vi "WildDrive.vi"(8 "Super Turn":bool, 9 "Turn":dbl, 11 "Speed":dbl) -> (1 "Right Side Power":dbl, 3 "Left Side Power":dbl)   [LabVIEW 2018]
panel:
  in  "Manual Feed Forward (Turn)":dbl
  in  "Manual Feed Forward (speed)":dbl
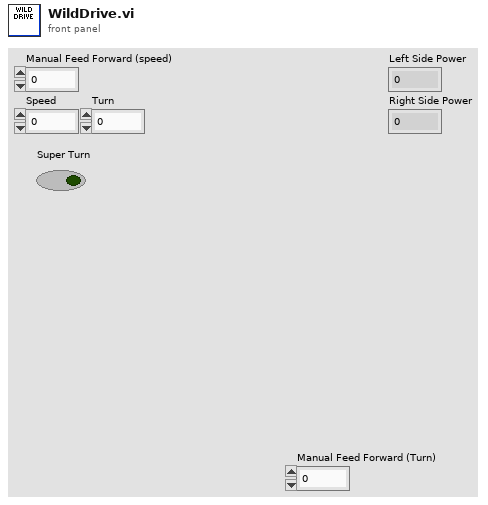
[diagram p1: front panel]
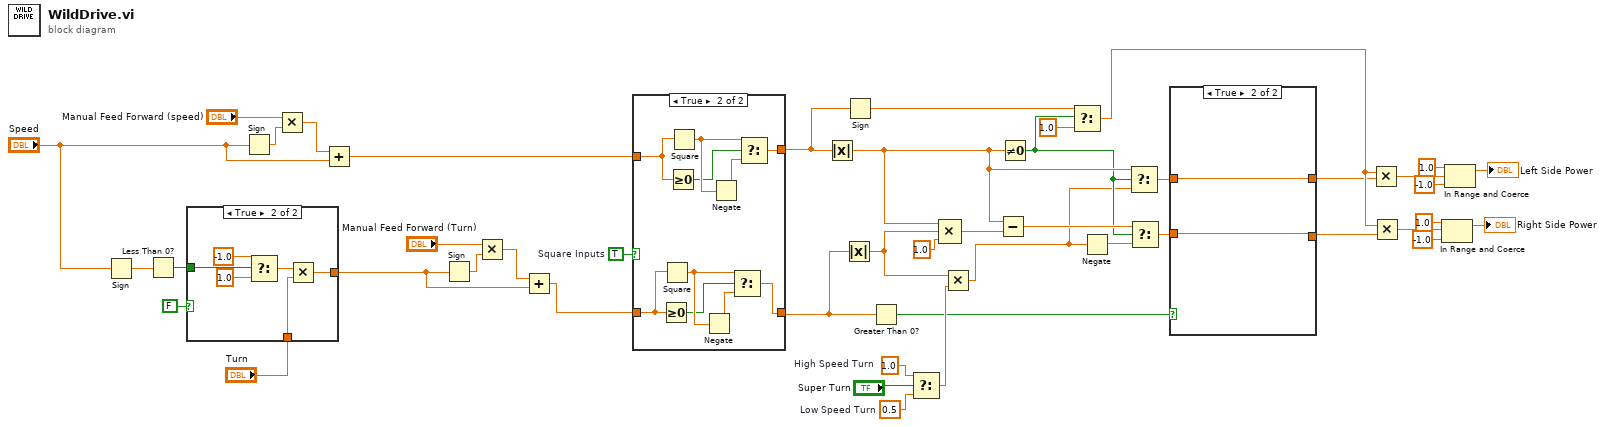
[diagram p0: block diagram]
diagram:
  w19 = 0.5  # Low Speed Turn
  w20 = 1.0  # High Speed Turn
  w35 = TRUE  # Square Inputs
  n1 = Sign(1:"Speed") -> (0:w41:dbl)
  n2 = Less Than 0?(x=w41) -> (x < 0?=w30:bool)
  n3 = case shown="True" FALSE {
    tunnel: "Turn" -> [w46 w49]
    tunnel: [w46 w48] -> w36
    tunnel: w30 -> [_ w47]
    frame False {
    }
    frame True {
      n4 = Select(t=-1.0, s=w47, f=1.0) -> (s? t:f=w50:dbl)
      n5 = Multiply(x=w50, y=w49) -> (x*y=w48:dbl)
    }
  }
  n6 = Sign(1:"Speed") -> (0:w43:dbl)
  n7 = Multiply(x="Manual Feed Forward (speed)", y=w43) -> (x*y=w44:dbl)
  n8 = Add(x=w44, y="Speed") -> (x+y=w33:dbl)
  n9 = Sign(1:w36) -> (0:w37:dbl)
  n10 = Multiply(x="Manual Feed Forward (Turn)", y=w37) -> (x*y=w38:dbl)
  n11 = Add(x=w38, y=w36) -> (x+y=w34:dbl)
  n12 = case shown="True" w35 {
    tunnel: w34 -> [w53 w64]
    tunnel: w33 -> [w54 w57]
    tunnel: [w54 w56] -> w32
    tunnel: [w53 w55] -> w26
    frame False {
    }
    frame True {
      n13 = Greater Or Equal To 0?(x=w64) -> (x >= 0?=w61:bool)
      n14 = Square(x=w64) -> (x^2=w63:dbl)
      n15 = Greater Or Equal To 0?(x=w57) -> (x >= 0?=w58:bool)
      n16 = Square(x=w57) -> (x^2=w60:dbl)
      n17 = Negate(x=w63) -> (-x=w62:dbl)
      n18 = Negate(x=w60) -> (-x=w59:dbl)
      n19 = Select(t=w63, s=w61, f=w62) -> (s? t:f=w55:dbl)
      n20 = Select(t=w60, s=w58, f=w59) -> (s? t:f=w56:dbl)
    }
  }
  n21 = Absolute Value(x=w32) -> (abs(x)=w25:dbl)
  n22 = Absolute Value(x=w26) -> (abs(x)=w22:dbl)
  n23 = Sign(1:w32) -> (0:w31:dbl)
  n24 = Greater Than 0?(x=w26) -> (x > 0?=w12:bool)
  n25 = Select(t=w20, s="Super Turn", f=w19) -> (s? t:f=w21:dbl)
  n26 = Compound Arithmetic op=MULTIPLY(w25, w22, 1.0 ("value")) -> (w23:dbl)
  n27 = Multiply(x=w22, y=w21) -> (x*y=w13:dbl)
  n28 = Subtract(x=w25, y=w23) -> (x-y=w16:dbl)
  n29 = Not Equal To 0?(x=w25) -> (x != 0?=w15:bool)
  n30 = Select(t=w31, s=w15, f=1.0) -> (s? t:f=w17:dbl)
  n31 = Negate(x=w13) -> (-x=w14:dbl)
  n32 = Select(t=w25, s=w15, f=w13) -> (s? t:f=w27:dbl)
  n33 = Select(t=w16, s=w15, f=w14) -> (s? t:f=w11:dbl)
  n34 = case shown="True" w12 {
    tunnel: w27 -> [w66 w68]
    tunnel: w11 -> [w65 w67]
    tunnel: [w65 w68] -> w1
    tunnel: [w66 w67] -> w10
    frame False {
    }
    frame True {
    }
  }
  n35 = Multiply(x=w17, y=w1) -> (x*y=w9:dbl)
  n36 = Multiply(x=w17, y=w10) -> (x*y=w6:dbl)
  n37 = In Range and Coerce(upper limit=1.0, x=w6, lower limit=-1.0) -> (coerced(x)=→"Right Side Power":dbl)  [unwired: 1 out]
  n38 = In Range and Coerce(upper limit=1.0, x=w9, lower limit=-1.0) -> (coerced(x)=→"Left Side Power":dbl)  [unwired: 1 out]
